vi "run_experiment_sCMOS_DAC_rough_working.vi"() -> ()   [LabVIEW 2015]
uses:
  <vilib>/DAQmx/write.llb/DAQmx Write (Digital Bool 1Line 1Point).vi
  <vilib>/DAQmx/write.llb/DAQmx Write (Analog 1D DBL 1Chan NSamp).vi
  <vilib>/DAQmx/read.llb/DAQmx Read (Analog 1D Wfm NChan NSamp).vi
  <vilib>/DAQmx/create/channels.llb/DAQmx Create Channel (DO-Digital Output).vi
  <vilib>/DAQmx/miscellaneous.llb/DAQmx Fill In Error Info.vi
  <vilib>/Analysis/1siggen.llb/Riffle Array (I32).vi
  <vilib>/addons/h5labview2/base/lib_path.vi
  <vilib>/addons/h5labview2/base/H5Equery.vi
  <vilib>/addons/h5labview2/dataset/H5Dwrite.llb/H5Dwrite.xnode
  <vilib>/addons/h5labview2/base/hid_t.ctl
  <vilib>/addons/h5labview2/dataset/H5D.lvlib
  <vilib>/addons/h5labview2/space/H5S.lvlib
  <vilib>/addons/h5labview2/file/H5F.lvlib
  <vilib>/Analysis/NI_AALBase.lvlib
panel:
  out "Stimulus Order":i32[](array[numeric])
  in  "Randomize":bool
  out "Stop Input":bool
  out "Numeric":i32
  out "DAC input":bool
  out "number of samples written per channel":u32
  out "error out 2":errorcluster
  out "temp .dcimg filepath":path
  out "Exposure":dbl
  out "V Width":i32
  out "H Width":i32
  out "Acquiring Frames":bool
  out "Frames Recorded":i32
  out "Display":T1(plugin-control)
  out "DAC Input":waveform(dbl)[](graph) caption="DAC Input Display"
  out "error out":errorcluster
  out "Current Stimulus Name":string
  out "Current Piezo Command":dynamicdata(graph)
  out "Current Stim Frames":i32
  out "Current Stim Duration":dbl
  out "Current Stimulus Save Path":path
  in  "Number Reps":dbl
  out "Experiment Path":path
  out "Timestamp":string
  out "Genotype":string
  out "Fly Name":string
  out "Experiment Name":string
  in  "Metadata Path":path
  out "Stimulus Files":path[](array[path])
  out "Num Stimuli":i32
  out "Protocol Name":string
  out "Protocol Rate":i32
  in  "Protocol Path":path
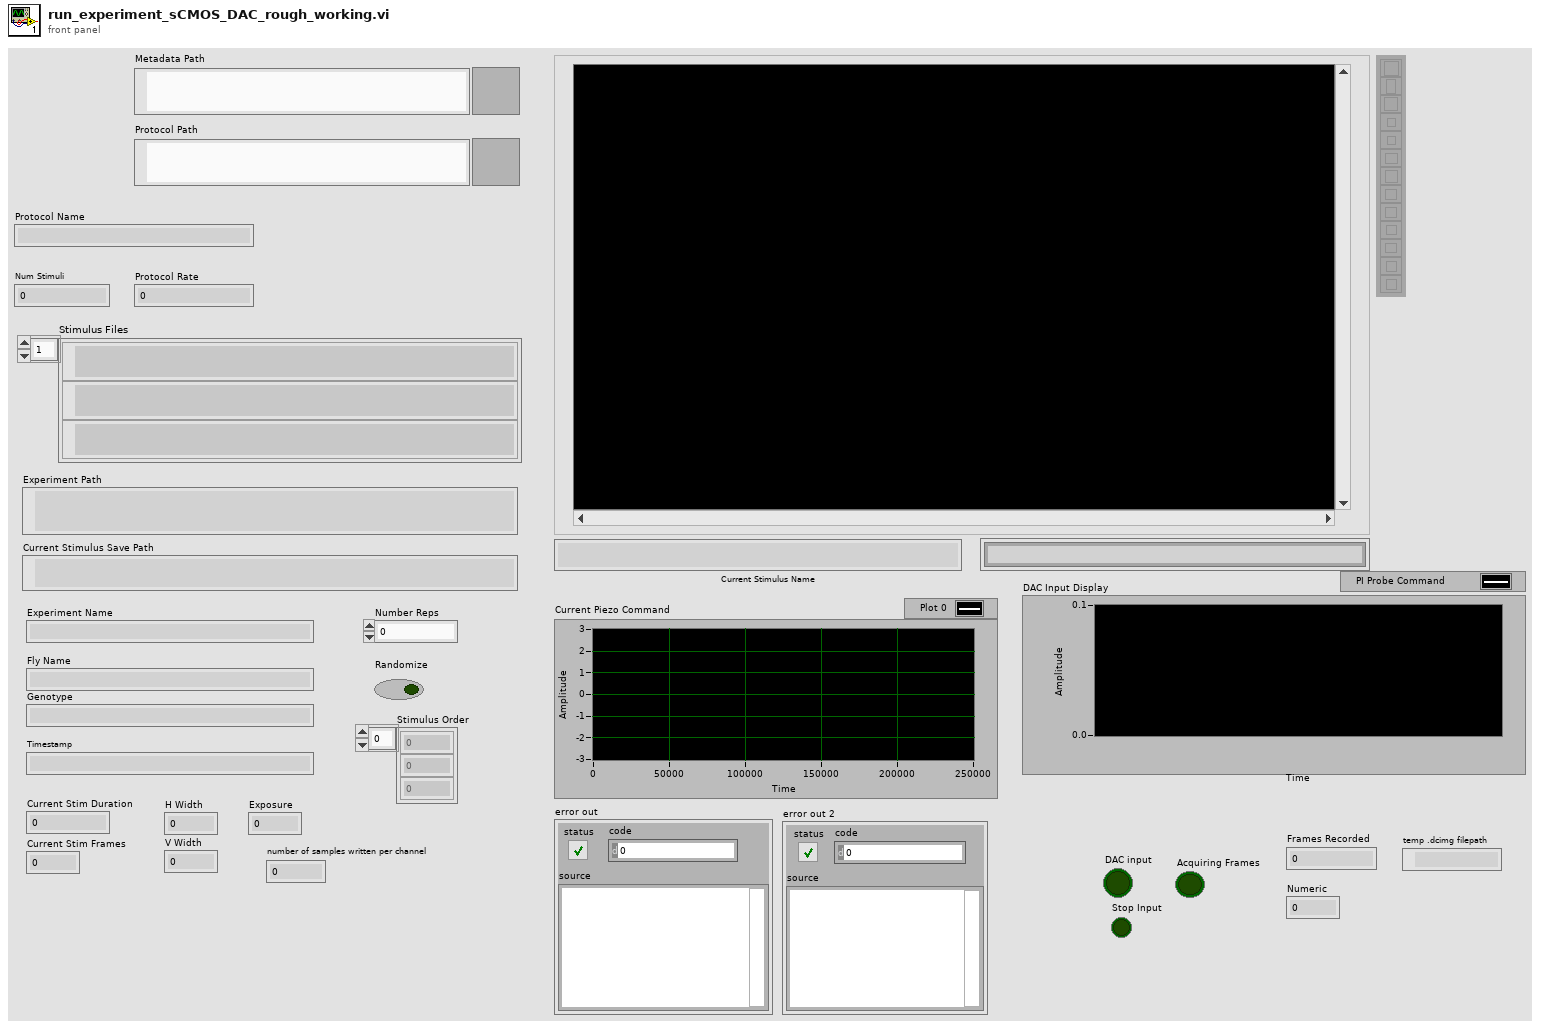
[diagram p1: front panel]
types:
  T1 = typedef "IMAQ Image.ctl" = refnum<image>
  T2 = cluster{"Value":i32, "Minimum":i32, "Maximum":i32, "Increment":i32}
  T3 = cluster{"Rows Per Strip":i32, "Photometric":i32, "Compression Type":i32}
  T4 = typedef "Image Type" = u32
  T5 = cluster{"height":u32, "width":u32, "datatype":u32}
  T6 = typedef "hid_t.ctl" = i32
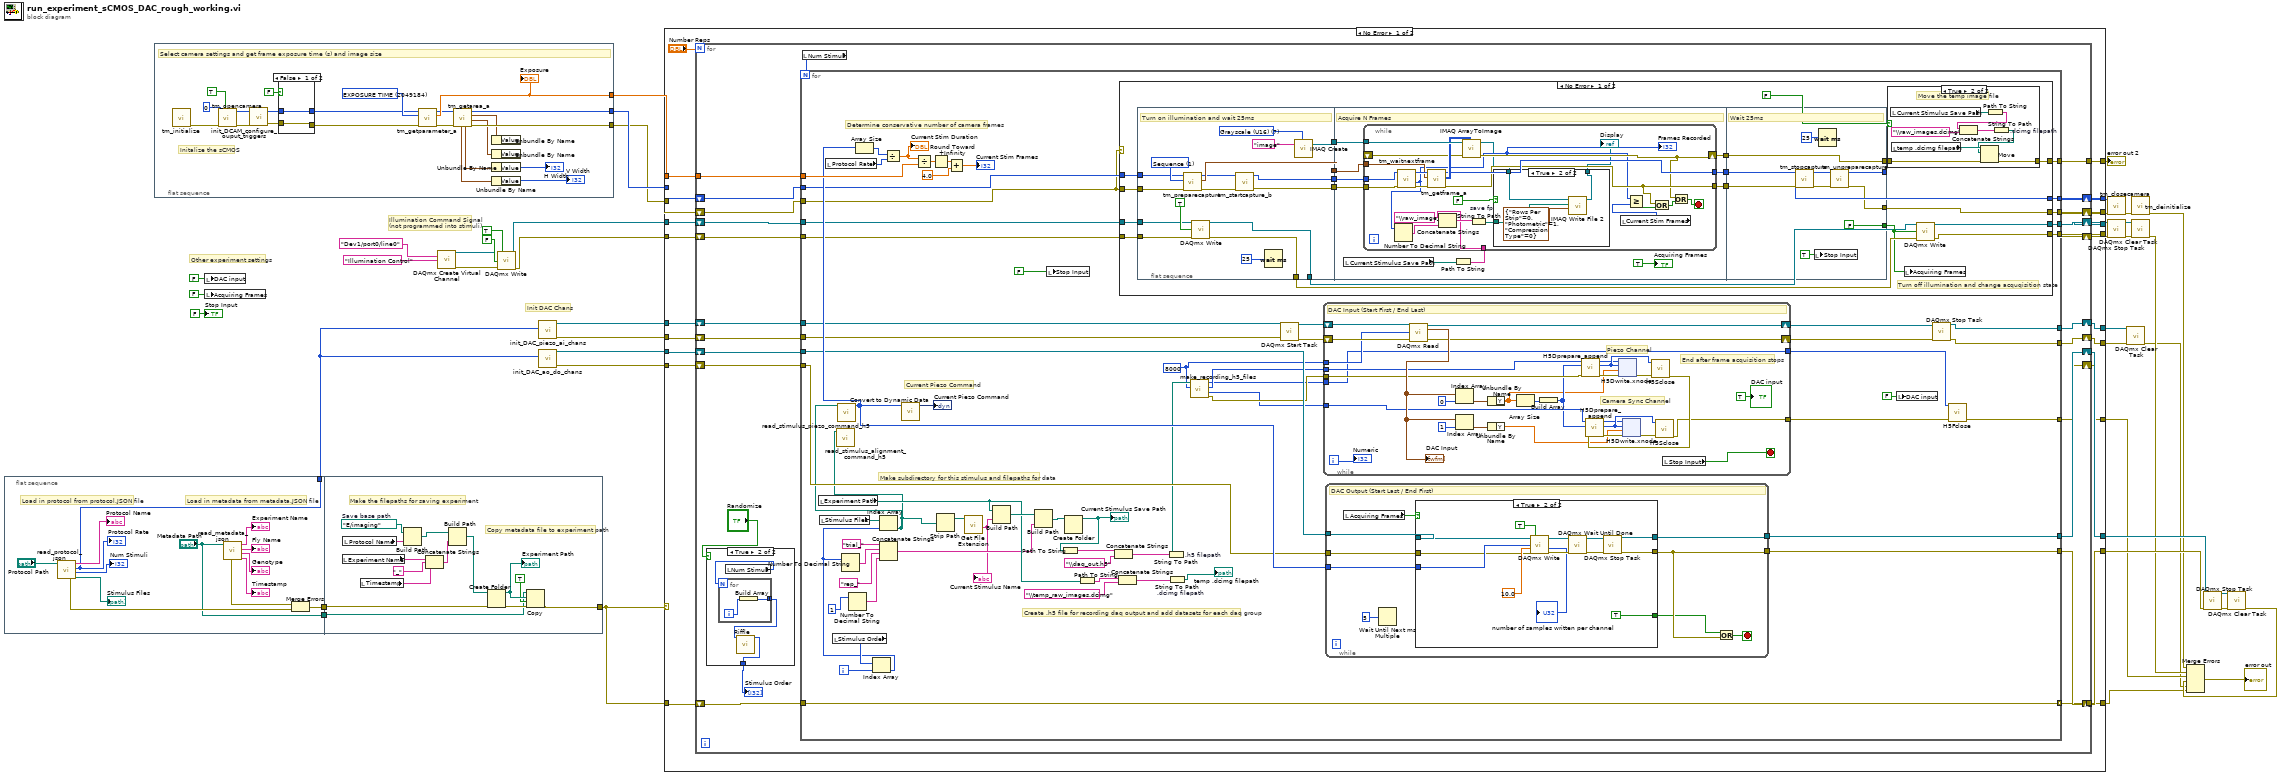
[diagram p0: block diagram]
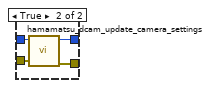
[diagram p2: hidden frame]
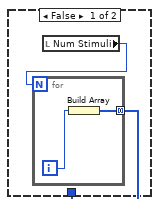
[diagram p3: hidden frame]
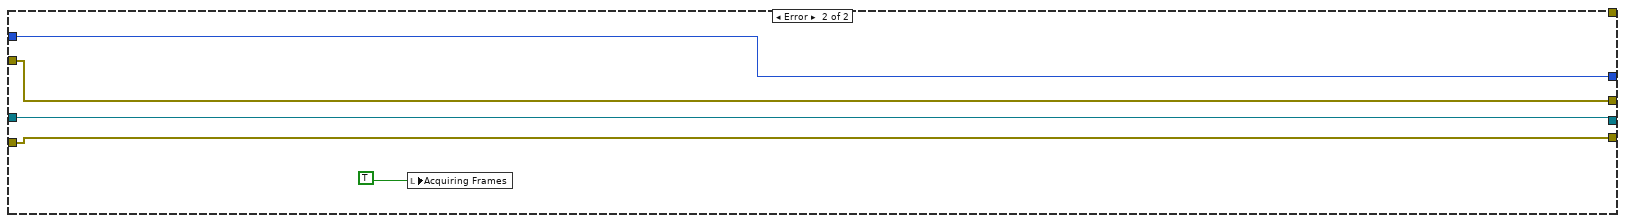
[diagram p6: hidden frame]
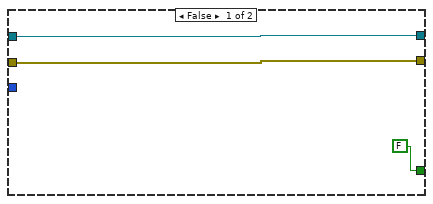
[diagram p7: hidden frame]
diagram:
  # "Other experiment settings"
  # "Init DAC Chans"
  # "Illumination Command Signal \n(not programmed into stimuli)"
  n1 = flat-sequence {
    tunnel: [w46] -> w40
    tunnel: [w47] -> w13
    tunnel: ["Metadata Path"] -> w12
    tunnel: w13 -> [w59]
    tunnel: w12 -> [w58]
    tunnel: [w57] -> w4
    frame #0 {
      # "Load in metadata from metadata.JSON file"
      # "Load in protocol from protocol.JSON file"
      n2 = call "read_protocol_json.vi"("Path"="Protocol Path") -> ("stims"=→"Stimulus Files":path[], "n_stims"=→"Num Stimuli":i32, "rate"=w46:i32, "protocol name"=→"Protocol Name":string, "error out"=w49:errorcluster)  [unwired: 6 in]
      "Protocol Rate" <- w46
      n3 = call "read_metadata_json.vi"("Path"="Metadata Path") -> ("exp_time"=→"Timestamp":string, "genotype"=→"Genotype":string, "fly_name"=→"Fly Name":string, "exp_ name"=→"Experiment Name":string, "error out"=w48:errorcluster)  [unwired: 6 in]
      n4 = Merge Errors(w48, w49) -> (w47:errorcluster)
    }
    frame #1 {
      w66 = path "E:/imaging"  # Save base path
      # "Copy metadata file to experiment path"
      # "Make the filepaths for saving experiment"
      n5 = local read "Experiment Name"() -> (w63:string)
      n6 = local read "Protocol Name"() -> (w65:string)
      n7 = local read "Timestamp"() -> (w61:string)
      n8 = Build Path(base path=w66, name or relative path=w65) -> (appended path=w64:path)
      n9 = Concatenate Strings(w63, "_", w61) -> (w60:string)
      n10 = Build Path(base path=w64, name or relative path=w60) -> (appended path=w67:path)
      n11 = Create Folder(path (use dialog)=w67, error in=w59) -> (created path=w70:path, error out=w69:errorcluster)  [unwired: 1 in, 1 out]
      "Experiment Path" <- w70
      n12 = Copy(8:w69, 9:TRUE ("overwrite (F)"), 10:w70, 11:w58) -> (0:w57:errorcluster)  [unwired: 1 in, 2 out]
    }
  }
  n13 = flat-sequence {
    tunnel: [w91] -> w10
    tunnel: [w90] -> w9
    tunnel: [w92] -> w11
    frame #0 {
      w84 = u32 2049184 items=["SENSOR MODE"=4212128, "CCD MODE"=4212384, "READOUT MODE"=4211872, "ACTIVE VIEW INDEX"=4343136, "BITS PER CHANNEL"=4342976, "IMAGE PIXEL TYPE"=4343296, "BINNING"=4215968, "EXPOSURE TIME"=2049184, "CONTRAST GAIN"=3163312, "CONTRAST OFFSET"=3163328, "LIGHT MODE"=2114720, "SENSITIVITY"=2114992, "PHOTON IMAGING MODE"=2115200, "HIGH DYNAMIC RANGE MODE"=3163360, "WHITE BALANCE"=3163568, "TEMPERATURE"=2115232, "TEMPERATURE TARGET"=2115264, "SENSOR COOLER FAN"=2115296, "LINEBUNDLE HEIGHT"=4212192, "MECHANICAL SHUTTER"=2115488, "BACK FOCUS POSITION"=8422304, "TRIGGER CONNECTOR"=1066432, "TRIGGER SOURCE"=1066144, "OUTPUT TRIGGER SOURCE"=1852576, "TRIGGER GLOBAL EXPOSURE"=2049680, "FIRST TRIGGER BEHAVIOR"=2049696, "CHANNEL SYNC"=1852352, "READOUT DIRECTION"=4211904, "PRE HSYNC COUNT"=1852704] ("Parameter")
      # "Initalize the sCMOS"
      # "Select camera settings and get frame exposure time (s) and image size"
      n14 = call <userlib>:"tm_initialize.vi"() -> ("error out"=w89:errorcluster)  [unwired: 8 in, 3 out]
      n15 = call <userlib>:"tm_opencamera.vi"("Force Open"=TRUE, "error in (no error)"=w89, "Camera Index"=0) -> ("error out"=w85:errorcluster, "Handle out"=w86:u32)  [unwired: 6 in, 1 out]
      n16 = call "init_DCAM_configure_ouput_triggers.vi"("error in (no error)"=w85, "Handle in"=w86) -> ("error out"=w72:errorcluster, "Handle out"=w73:u32)  [unwired: 2 in]
      n17 = case shown="False" FALSE {
        tunnel: [w93 w98] -> w75
        tunnel: [w94 w97] -> w74
        tunnel: w73 -> [w94 w96]
        tunnel: w72 -> [w93 w95]
        frame False {
        }
        frame True {
          n18 = call "hamamatsu_dcam_update_camera_settings.vi"("error in (no error)"=w95, "Handle in"=w96) -> ("error out"=w98:errorcluster, "Handle out"=w97:u32)  [unwired: 6 in]
        }
      }
      n19 = call <userlib>:"tm_getparameter_a.vi"("error in (no error)"=w75, "Parameter"=w84, "Handle in"=w74) -> ("error out"=w79:errorcluster, "Value out"=w92:dbl, "Handle out"=w78:u32)  [unwired: 6 in]
      "Exposure" <- w92
      n20 = call <userlib>:"tm_getarea_a.vi"("error in (no error)"=w79, "Handle in"=w78) -> ("error out"=w90:errorcluster, "V Offset"=w82:T2, "H Offset"=w83:T2, "Handle out"=w91:u32, "H Width"=w81:T2, "V Width"=w80:T2)  [unwired: 4 in]
      n21 = Unbundle By Name(w83) -> ()  [unwired: 1 out]
      n22 = Unbundle By Name(w82) -> ()  [unwired: 1 out]
      n23 = Unbundle By Name(w81) -> ("Value"=→"H Width":i32)
      n24 = Unbundle By Name(w80) -> ("Value"=→"V Width":i32)
    }
  }
  n25 = local write "DAC input"(FALSE ("DAC input")) -> ()
  n26 = local write "Acquiring Frames"(FALSE ("Acquiring Frames")) -> ()
  n27 = call-poly <vilib>:"DAQmx Create Virtual Channel.vi"("lines"=tag "Dev1/port0/line0" ("DAQmx Physical Channel"), "name to assign"="Illumination Control") -> ("task out"=w7:refnum<k21>, "error out"=w6:errorcluster)  [unwired: 12 in]
  n28 = call-poly <vilib>:"DAQmx Write.vi"("task/channels in"=w7, "auto start"=TRUE, "data"=FALSE, "error in"=w6) -> ("task out"=w19:refnum<k21>, "error out"=w18:errorcluster)  [unwired: 9 in, 1 out]
  n29 = call "init_DAC_piezo_ai_chans.vi"("Sample Rate"=w40) -> ("error out"=w16:errorcluster, "Refnum out"=w17:refnum<k21>)  [unwired: 8 in, 1 out]
  n30 = call "init_DAC_ao_do_chans.vi"("Rate"=w40) -> ("error out"=w14:errorcluster, "AO Out"=w15:refnum<k21>)  [unwired: 8 in, 1 out]
  n31 = case shown="No Error" w4 {
    tunnel: w11 -> [w120 _]
    tunnel: w10 -> [w119 w415]
    tunnel: w9 -> [w118 w414]
    tunnel: [w112 _] -> w27
    tunnel: [w111 _] -> w28
    tunnel: [w117 _] -> w31
    tunnel: [w116 _] -> w32
    tunnel: [w115 w414] -> w24
    tunnel: [w114 w415] -> w23
    tunnel: [w113 _] -> w30
    tunnel: [w110 _] -> w22
    tunnel: [w109 _] -> w21
    tunnel: w19 -> [w108 _]
    tunnel: w18 -> [w107 _]
    tunnel: w17 -> [w106 _]
    tunnel: w16 -> [w105 _]
    tunnel: w15 -> [w104 _]
    tunnel: w14 -> [w103 _]
    tunnel: [w102 _] -> w5
    tunnel: w4 -> [w101 _]
    tunnel: [w100 _] -> w3
    frame No Error {
      n32 = for {
        N: "Number Reps" -> [_]
        tunnel: w120 -> [w144]
        tunnel: [w126] -> w102
        tunnel: [w124] -> w100
        shift-right: [w138] -> w114
        shift-left: w119 -> [w143]
        shift-right: [w139] -> w115
        shift-left: w118 -> [w142]
        shift-right: [w136] -> w112
        shift-left: w108 -> [w132]
        shift-right: [w135] -> w111
        shift-left: w107 -> [w131]
        shift-right: [w133] -> w109
        shift-left: w106 -> [w130]
        shift-right: [w134] -> w110
        shift-left: w105 -> [w129]
        shift-right: [w140] -> w116
        shift-left: w104 -> [w128]
        shift-right: [w137] -> w113
        shift-left: w103 -> [w127]
        shift-right: [w141] -> w117
        shift-left: w101 -> [w125]
        n33 = case shown="True" "Randomize" {
          tunnel: [w145 w149] -> w121
          frame False {
            n34 = local read "Num Stimuli"() -> (w146:i32)
            n35 = for {
              N: w146 -> [_]
              tunnel: [w148] -> w145 mode=concatenating
              i -> [w147]
              n36 = Build Array(w147) -> (w148:i32[])
            }
          }
          frame True {
            n37 = local read "Num Stimuli"() -> (w151:i32)
            n38 = for {
              N: w151 -> [_]
              tunnel: [w152] -> w150 mode=concatenating
              i -> [w153]
              n39 = Build Array(w153) -> (w152:i32[])
            }
            n40 = call-poly <vilib>:"Riffle.vi"("X"=w150) -> ("Riffled {X}"=w149:i32[])  [unwired: 8 in, 2 out]
          }
        }
        "Stimulus Order" <- w121
        n41 = local read "Num Stimuli"() -> (w123:i32)
        n42 = for {
          N: w123 -> [_]
          tunnel: w144 -> [w214]
          tunnel: w143 -> [w192]
          tunnel: w142 -> [w158]
          tunnel: [w209] -> w141
          tunnel: [w208] -> w140
          tunnel: [w175] -> w139
          tunnel: [w176] -> w138
          tunnel: [w204] -> w137
          tunnel: [w200] -> w136
          tunnel: [w199] -> w135
          tunnel: [w198] -> w134
          tunnel: [w197] -> w133
          tunnel: w132 -> [w177]
          tunnel: w131 -> [w178]
          tunnel: w130 -> [w196]
          tunnel: w129 -> [w195]
          tunnel: w128 -> [w194]
          tunnel: w127 -> [w193]
          tunnel: [w169] -> w126
          tunnel: w125 -> [w168]
          tunnel: [w168] -> w124 mode=indexing
          i -> [w155]
          w161 = 8000 ("dimension size")
          # "Create .h5 file for recording daq output and add datasets for each daq group"
          # "Current Piezo Command"
          # "Determine conservative number of camera frames"
          # "Make subdirectory for this stimulus and filepaths for data"
          n43 = local read "Experiment Path"() -> (w182:path)
          n44 = local read "Stimulus Files"() -> (w218:path[])
          n45 = local read "Protocol Rate"() -> (w171:i32)
          n46 = local read "Stimulus Order"() -> (w156:i32[])
          n47 = Number To Decimal String(number=i16 1 ("width (-)")) -> (decimal integer string=w216:string)  [unwired: 1 in]
          n48 = Index Array(array=w156, index=w155) -> (element=w154:i32)
          n49 = Number To Decimal String(number=w154) -> (decimal integer string=w220:string)  [unwired: 1 in]
          n50 = Concatenate Strings("trial_", w220, "rep_", w216) -> (w180:string)
          n51 = Index Array(array=w218, index=w154) -> (element=w181:path)
          n52 = call "read_stimulus_alignment_command_h5.vi"("Path"=w181) -> ()  [unwired: 9 in, 2 out]
          n53 = call "read_stimulus_piezo_command_h5.vi"("Path"=w181) -> ("stimulus"=w203:i32[])  [unwired: 9 in, 1 out]
          n54 = Array Size(array=w203) -> (size(s)=w172:i32)
          n55 = Divide(x=w172, y=w171) -> (x/y=w170:dbl)
          "Current Stim Duration" <- w170
          n56 = call "Convert to Dynamic Data"("Array"=w203) -> ("Dynamic Data Type"=→"Current Piezo Command":dynamicdata)  [unwired: 3 in]
          n57 = Divide(x=w170, y=w214) -> (x/y=w213:dbl)
          n58 = Round Toward +Infinity(x=w213) -> (ceil(x): smallest int >= x=w212:dbl)
          n59 = Strip Path(path=w181) -> (stripped path=w186:path)  [unwired: 1 out]
          n60 = Add(x=w212, y=4.0) -> (x+y=→"Current Stim Frames":dbl)
          n61 = call <vilib>:"Get File Extension.vi"("file"=w186) -> ("filename without extension"=w159:string)  [unwired: 6 in, 4 out]
          "Current Stimulus Name" <- w159
          n62 = Build Path(base path=w182, name or relative path=w159) -> (appended path=w187:path)
          n63 = Build Path(base path=w187, name or relative path=w180) -> (appended path=w188:path)
          n64 = local write "Stop Input"(FALSE ("Stop Input")) -> ()
          n65 = Create Folder(path (use dialog)=w188) -> (created path=w174:path)  [unwired: 2 in, 2 out]
          "Current Stimulus Save Path" <- w174
          n66 = Path To String(path=w174) -> (string=w184:string)
          n67 = Path To String(path=w182) -> (string=w189:string)
          n68 = Concatenate Strings(w184, "\\daq_out.h5" ("string")) -> (w183:string)
          n69 = Concatenate Strings(w189, "\\temp_raw_images.dcimg" ("string")) -> (w191:string)
          n70 = case shown="No Error" w158 {
            tunnel: [w234 w319] -> w200
            tunnel: [w233 w318] -> w199
            tunnel: w192 -> [w232 w321]
            tunnel: w158 -> [w231 w320]
            tunnel: w178 -> [w230 w318]
            tunnel: w177 -> [w229 w319]
            tunnel: [w226 w321] -> w176
            tunnel: [w225 w320] -> w175
            tunnel: [w223 _] -> w169
            frame No Error {
              # "Turn off illumination and change acquqisition state"
              n71 = flat-sequence {
                tunnel: [w251] -> w241
                tunnel: [w263] -> w240
                tunnel: [w252] -> w239
                tunnel: [w260] -> w238
                tunnel: w232 -> [w265]
                tunnel: w231 -> [w264]
                tunnel: w230 -> [w258]
                tunnel: w229 -> [w257]
                tunnel: [w256] -> w228
                tunnel: [w255] -> w227
                tunnel: w241 -> [w276]
                tunnel: w240 -> [w275]
                tunnel: w239 -> [w274]
                tunnel: [w273] -> w237
                tunnel: [w272] -> w236
                tunnel: w238 -> [w271]
                tunnel: [w270] -> w235
                tunnel: [FALSE] -> w221
                tunnel: w237 -> [w312]
                tunnel: w236 -> [w313]
                tunnel: [w308] -> w225
                tunnel: [w310] -> w226
                tunnel: w235 -> [w314]
                tunnel: [w314] -> w224
                frame #0 {
                  w262 = T4 7 items=["Grayscale (U8)", "Grayscale (I16)", "Grayscale (SGL)", "Complex (CSG)", "RGB (U32)", "HSL (U32)", "RGB (U64)", "Grayscale (U16)"] ("Image Type")
                  w266 = 1 items=["Snap", "Sequence"] ("Capture mode")
                  # "Turn on illumination and wait 25ms"
                  n72 = call <userlib>:"tm_preparecapture.vi"("error in (no error)"=w264, "Capture mode"=w266, "Handle in"=w265) -> ("error out"=w254:errorcluster, "Buffer Info"=w263:T5, "Handle out"=w253:u32)  [unwired: 5 in, 1 out]
                  n73 = call-poly <vilib>:"DAQmx Write.vi"("task/channels in"=w257, "data"=TRUE, "error in"=w258) -> ("task out"=w256:refnum<k21>, "error out"=w255:errorcluster)  [unwired: 10 in, 1 out]
                  n74 = call <userlib>:"tm_startcapture_b.vi"("error in (no error)"=w254, "Handle in"=w253) -> ("error out"=w251:errorcluster, "Handle out"=w252:u32)  [unwired: 8 in]
                  n75 = Wait (ms)(milliseconds to wait=u32 25) -> ()  [unwired: 1 out]
                  n76 = call "IMAQ Create"("Image Name"="image", "Image Type"=w262) -> ("New Image"=w260:T1)  [unwired: 3 in, 1 out]
                }
                frame #1 {
                  # "Acquire N Frames"
                  n77 = local read "Current Stimulus Save Path"() -> (w269:path)
                  n78 = Path To String(path=w269) -> (string=w268:string)
                  n79 = while {
                    tunnel: w276 -> [w299]
                    tunnel: w275 -> [w298]
                    tunnel: w274 -> [w297]
                    tunnel: [w292] -> w273
                    tunnel: [w290] -> w272
                    tunnel: w271 -> [w295]
                    shift-right: [w289] -> w270
                    shift-left: _ -> [w293]
                    tunnel: w268 -> [w282]
                    stop <- w287 stop-if-true
                    n80 = call <userlib>:"tm_waitnextframe.vi"("error in (no error)"=w299, "Handle in"=w297) -> ("error out"=w301:errorcluster, "Frame Count"=w286:i32, "Handle out"=w300:u32)  [unwired: 6 in, 1 out]
                    "Frames Recorded" <- w286
                    n81 = Number To Decimal String(number=w286) -> (decimal integer string=w285:string)  [unwired: 1 in]
                    n82 = call <userlib>:"tm_getframe_a.vi"("error in (no error)"=w301, "Buffer Info"=w298, "Handle in"=w300) -> ("error out"=w290:errorcluster, "Data 16"=w294:u16[][], "Handle out"=w292:u32)  [unwired: 4 in, 2 out]
                    n83 = Concatenate Strings(w282, "\\raw_image_" ("string"), w285) -> (w283:string)
                    n84 = call "IMAQ ArrayToImage"("Image Pixels (U16)"=w294, "error in (no error)"=w293, "Image"=w295) -> ("error out"=w289:errorcluster, "Image Out"=w280:T1)  [unwired: 7 in]
                    n85 = String To Path "save fp"(string=w283) -> (path=w279:path)
                    n86 = case shown="True" FALSE {
                      tunnel: w280 -> [w302 w306]
                      tunnel: w279 -> [_ w305]
                      tunnel: [w302 w303] -> w278
                      frame False {
                      }
                      frame True {
                        n87 = call-poly "IMAQ Write File 2"("TIFF Options"=T3 {"Rows Per Strip"=0, "Photometric"=1, "Compression Type"=0}, "File Path"=w305, "Image"=w306) -> ("Image Out (duplicate)"=w303:T1)  [unwired: 7 in, 1 out]
                      }
                    }
                    "Display" <- w278
                    n88 = local read "Current Stim Frames"() -> (w296:i32)
                    n89 = Greater Or Equal?(x=w286, y=w296) -> (x >= y?=w291:bool)
                    n90 = Or(x=w290, y=w291) -> (x .or. y?=w288:bool)
                    n91 = Or(x=w289, y=w288) -> (x .or. y?=w287:bool)
                  }
                  "Acquiring Frames" <- TRUE
                }
                frame #2 {
                  # "Wait 25ms"
                  n92 = call <userlib>:"tm_stopcapture.vi"("error in (no error)"=w313, "Handle in"=w312) -> ("error out"=w309:errorcluster, "Handle out"=w311:u32)  [unwired: 8 in]
                  n93 = local write "Stop Input"(TRUE ("Stop Input")) -> ()
                  n94 = Wait (ms)(milliseconds to wait=u32 25) -> ()  [unwired: 1 out]
                  n95 = call <userlib>:"tm_unpreparecapture.vi"("error in (no error)"=w309, "Handle in"=w311) -> ("error out"=w308:errorcluster, "Handle out"=w310:u32)  [unwired: 8 in]
                }
              }
              n96 = case shown="True" FALSE {
                tunnel: w224 -> [w242 w244]
                tunnel: [w242 w243] -> w223
                frame False {
                }
                frame True {
                  # "Move the temp image file"
                  n97 = local read "Current Stimulus Save Path"() -> (w246:path)
                  n98 = local read "temp .dcimg filepath"() -> (w250:path)
                  n99 = Path To String(path=w246) -> (string=w247:string)
                  n100 = Concatenate Strings(w247, "\\raw_images.dcimg" ("string")) -> (w249:string)
                  n101 = String To Path ".dcimg filepath"(string=w249) -> (path=w245:path)
                  n102 = Move(source path=w250, error in=w244, 10:w245) -> (error out=w243:errorcluster)  [unwired: 2 in, 2 out]
                }
              }
              n103 = local write "Acquiring Frames"(w221) -> ()
              n104 = call-poly <vilib>:"DAQmx Write.vi"("task/channels in"=w228, "data"=w221, "error in"=w227) -> ("task out"=w234:refnum<k21>, "error out"=w233:errorcluster)  [unwired: 10 in, 1 out]
            }
            frame Error {
              n105 = local write "Acquiring Frames"(TRUE ("Acquiring Frames")) -> ()
            }
          }
          n106 = String To Path ".h5 filepath"(string=w183) -> (path=w167:path)
          n107 = String To Path ".dcimg filepath"(string=w191) -> (path=→"temp .dcimg filepath":path)
          n108 = call "make_recording_h5_files.vi"("write/append size"=w161, "Path"=w167) -> ("error out"=w166:errorcluster, "Camera Dataset"=w165:T6, "Piezo Dataset"=w164:T6, "ref out"=w162:T6)  [unwired: 6 in]
          n109 = call <vilib>:"DAQmx Start Task.vi"("task/channels in"=w196, "error in"=w195) -> ("task out"=w207:refnum<k21>, "error out"=w206:errorcluster)  [unwired: 12 in]
          n110 = while {
            tunnel: w166 -> [w364]
            tunnel: [w355] -> w205
            shift-right: [w356] -> w202
            shift-left: w207 -> [w377]
            shift-right: [w354] -> w201
            shift-left: w206 -> [w376]
            tunnel: w161 -> [w353]
            tunnel: w165 -> [w359]
            tunnel: w164 -> [w365]
            tunnel: [w351] -> w163
            tunnel: w162 -> [w351]
            i -> [w352]
            stop <- w349 stop-if-true
            # "End after frame acquisition stops"
            # "Camera Sync Channel"
            # "Piezo Channel"
            # "DAC Input (Start First / End Last)"
            n111 = call-poly <vilib>:"DAQmx Read.vi"("task/channels in"=w377, "number of samples per channel"=w353, "error in"=w376) -> ("task out"=w356:refnum<k21>, "data"=w371:waveform(dbl)[], "error out"=w354:errorcluster)  [unwired: 10 in]
            "DAC Input" <- w371
            n112 = Index Array(array=w371, index=0) -> (element=w375:waveform(dbl))
            n113 = Index Array(array=w371, index=1) -> (element=w373:waveform(dbl))
            n114 = Unbundle By Name(w375) -> ("Y"=w347:dbl[])
            n115 = Unbundle By Name(w373) -> ("Y"=w348:dbl[])
            n116 = Array Size(array=w347) -> (size(s)=w366:i32)
            n117 = Build Array(w366) -> (w358:i32[])
            n118 = call <vilib>:"H5Dprepare_append.vi"("error in (no error)"=w364, "append dims"=w358, "dset in"=w365) -> ("error out"=w367:errorcluster, "space out"=w370:T6, "dset out"=w368:T6)  [unwired: 6 in]
            n119 = xnode "H5Dwrite.xnode"("error in (no error)"=w367, "data"=w347, "file space"=w370, "ref in"=w368) -> ("error out"=w369:errorcluster)  [unwired: 3 in, 2 out]
            n120 = call <vilib>:"H5Sclose.vi"("error in (no error)"=w369, "space in"=w370) -> ("error out"=w357:errorcluster)  [unwired: 9 in]
            n121 = call <vilib>:"H5Dprepare_append.vi"("error in (no error)"=w357, "append dims"=w358, "dset in"=w359) -> ("error out"=w360:errorcluster, "space out"=w363:T6, "dset out"=w361:T6)  [unwired: 6 in]
            n122 = xnode "H5Dwrite.xnode"("error in (no error)"=w360, "data"=w348, "file space"=w363, "ref in"=w361) -> ("error out"=w362:errorcluster)  [unwired: 3 in, 2 out]
            n123 = call <vilib>:"H5Sclose.vi"("error in (no error)"=w362, "space in"=w363) -> ("error out"=w355:errorcluster)  [unwired: 9 in]
            n124 = local read "Stop Input"() -> (w349:bool)
            "DAC input" <- TRUE ("DAC input")
            "Numeric" <- w352
          }
          n125 = while {
            tunnel: w203 -> [w329]
            tunnel: w194 -> [w326]
            tunnel: [w327] -> w208
            tunnel: [w323] -> w209
            tunnel: w193 -> [w325]
            stop <- w324 stop-if-true
            # "DAC Output (Start Last / End First)"
            n126 = local read "Acquiring Frames"() -> (w330:bool)
            n127 = Wait Until Next ms Multiple(millisecond multiple=u32 5) -> ()  [unwired: 1 out]
            n128 = case shown="True" w330 {
              tunnel: w325 -> [w332 w340]
              tunnel: w326 -> [w333 w341]
              tunnel: w329 -> [_ w343]
              tunnel: [w333 w345] -> w327
              tunnel: [w332 w344] -> w323
              tunnel: [FALSE ("Stop Input") TRUE ("Stop Input")] -> w322
              frame False {
              }
              frame True {
                n129 = call-poly <vilib>:"DAQmx Write.vi"("task/channels in"=w341, "auto start"=TRUE, "data"=w343, "timeout"=10.0, "error in"=w340) -> ("task out"=w337:refnum<k21>, "number of samples written per channel"=→"number of samples written per channel":u32, "error out"=w336:errorcluster)  [unwired: 8 in]
                n130 = call <vilib>:"DAQmx Wait Until Done.vi"("task/channels in"=w337, "error in"=w336) -> ("task out"=w339:refnum<k21>, "error out"=w338:errorcluster)  [unwired: 12 in]
                n131 = call <vilib>:"DAQmx Stop Task.vi"("task/channels in"=w339, "error in"=w338) -> ("task out"=w345:refnum<k21>, "error out"=w344:errorcluster)  [unwired: 12 in]
              }
            }
            n132 = Or(x=w322, y=w323) -> (x .or. y?=w324:bool)
          }
          n133 = local write "DAC input"(FALSE ("DAC input")) -> ()
          n134 = call <vilib>:"DAQmx Stop Task.vi"("task/channels in"=w202, "error in"=w201) -> ("task out"=w197:refnum<k21>, "error out"=w198:errorcluster)  [unwired: 12 in]
          n135 = call <vilib>:"H5Fclose.vi"("error in (no error)"=w205, "ref"=w163) -> ("error out"=w204:errorcluster)  [unwired: 9 in]
        }
      }
    }
    frame Error {
    }
  }
  "error out 2" <- w5
  n136 = call <userlib>:"tm_closecamera.vi"("error in (no error)"=w24, "Handle in"=w23) -> ("error out"=w35:errorcluster)  [unwired: 9 in]
  n137 = call <vilib>:"DAQmx Stop Task.vi"("task/channels in"=w27, "error in"=w28) -> ("task out"=w37:refnum<k21>, "error out"=w36:errorcluster)  [unwired: 12 in]
  n138 = call <vilib>:"DAQmx Clear Task.vi"("task in"=w21, "error in"=w22) -> ("error out"=w20:errorcluster)  [unwired: 13 in]
  n139 = call <userlib>:"tm_deinitialize.vi"("error in (no error)"=w35) -> ("error out"=w25:errorcluster)  [unwired: 10 in]
  n140 = call <vilib>:"DAQmx Clear Task.vi"("task in"=w37, "error in"=w36) -> ("error out"=w26:errorcluster)  [unwired: 13 in]
  n141 = call <vilib>:"DAQmx Stop Task.vi"("task/channels in"=w32, "error in"=w31) -> ("task out"=w34:refnum<k21>, "error out"=w33:errorcluster)  [unwired: 12 in]
  n142 = call <vilib>:"DAQmx Clear Task.vi"("task in"=w34, "error in"=w33) -> ("error out"=w29:errorcluster)  [unwired: 13 in]
  n143 = Merge Errors(w25, w26, w30, w29, w20, w3) -> (→"error out":errorcluster)
  "Stop Input" <- FALSE ("Stop Input")
